vi "syncMaxWithAverage.vi"(6 "enable":bool, 8 "inputValid":bool, 9 "syncPoint":u16, 10 "syncAverageBand":u16=2 caption="syncAverageBand (2^n)", 11 "input":cluster{"index":u16, "data":i16}) -> (0 "outputValid":bool, 3 "waveMaxAvg":fxp<+/-,24,16>)   [LabVIEW 2016]
uses:
  <instrlib>/_niInstr/Basic Elements/v1/FPGA/niInstr Basic Elements v1 FPGA.lvlib
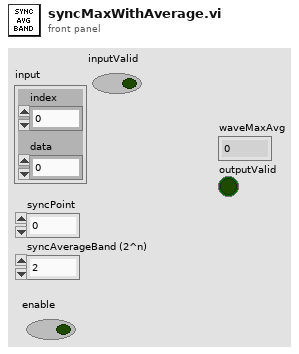
[diagram p1: front panel]
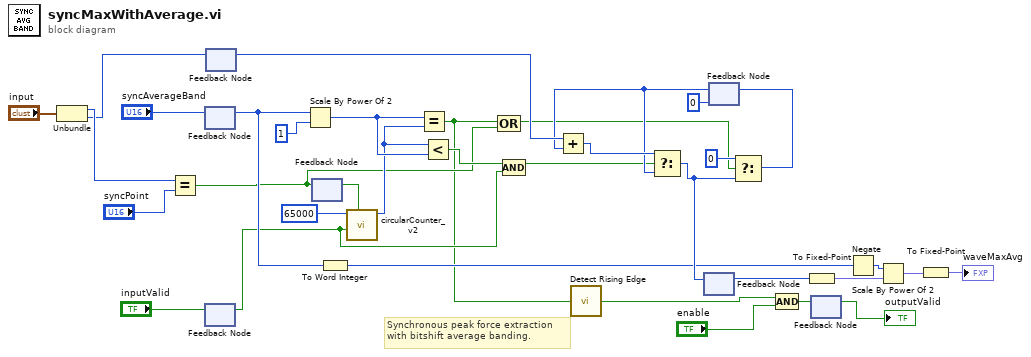
[diagram p0: block diagram]
diagram:
  # "Synchronous peak force extraction\nwith bitshift average banding."
  n1 = Unbundle("input") -> ("index"=w10:u16, "data"=w9:i16)
  n2 = Equal?(x=w10, y="syncPoint") -> (x = y?=w3:bool)
  n3 = feedback #1() -> (w23:u16)  [unwired: 1 in]
  n4 = feedback-in #1("syncAverageBand") -> ()
  n5 = feedback-in #2("inputValid") -> ()
  n6 = feedback #2() -> (w6:bool)  [unwired: 1 in]
  n7 = feedback #3() -> (w22:i16)  [unwired: 1 in]
  n8 = feedback-in #3(w9) -> ()
  n9 = Scale By Power Of 2(n=w23, x=i16 1) -> (x*2^n=w26:i16)
  n10 = feedback #4() -> (w4:bool)  [unwired: 1 in]
  n11 = feedback-in #4(w3) -> ()
  n12 = To Word Integer(number=w23) -> (16bit integer=w28:i16)
  n13 = call "circularCounter_v2.vi"("reset"=w4, "doStep"=w6, "maxCount"=u16 65000) -> ("index"=w24:u16)  [unwired: 5 in, 3 out]
  n14 = Equal?(x=w26, y=w24) -> (x = y?=w2:bool)
  n15 = Less?(x=w24, y=w26) -> (x < y?=w34:bool)
  n16 = Compound Arithmetic op=OR(w2, w3) -> (w5:bool)
  n17 = Compound Arithmetic op=AND(w34, w6) -> (w8:bool)
  n18 = call <instrlib>:"Detect Rising Edge.vi"("signal"=w2) -> ("edge detected"=w1:bool)  [unwired: 14 in]
  n19 = feedback #5() -> (w18:i32)  [unwired: 1 in]
  n20 = feedback #6(0 ("t")) -> (w21:i32)
  n21 = Add(x=w22, y=w21) -> (x+y=w33:i32)
  n22 = Select(t=w33, s=w8, f=w21) -> (s? t:f=w30:i32)
  n23 = feedback-in #5(w30) -> ()
  n24 = Select(t=0, s=w5, f=w30) -> (s? t:f=w20:i32)
  n25 = feedback-in #6(w20) -> ()
  n26 = Compound Arithmetic op=AND(w1, "enable") -> (w35:bool)
  n27 = To Fixed-Point(number=w18) -> (fixed-point=w16:fxp<+/-,36,28>)  [unwired: 1 in]
  n28 = feedback #7() -> (→"outputValid":bool)  [unwired: 1 in]
  n29 = feedback-in #7(w35) -> ()
  n30 = Negate(x=w28) -> (-x=w29:i16)
  n31 = Scale By Power Of 2(n=w29, x=w16) -> (x*2^n=w15:fxp<+/-,36,28>)
  n32 = To Fixed-Point(number=w15) -> (fixed-point=→"waveMaxAvg":fxp<+/-,24,16>)  [unwired: 1 in]
